vi "LiveMode.vi"() -> ()   [LabVIEW 2019]
uses:
  Data/GetPixelData16.vi
panel:
  in  "Centre AOI":bool
  in  "AOI Width":i64=2560
  in  "AOI Height":i64=2160
  out "Ready":bool
  in  "Run":bool
  in  "error":errorcluster
  out "Pixel Encoding":string
  out "Intensity Graph":u16[][](graph)
  out "AOIStride":i64
  in  "PreAmp":string(combo)="16-bit (low noise & high well capacity)"
  out "PixelData":u16[](array[numeric])
  out "ByteData":u8[](array[numeric])
  in  "ExposureTime":dbl=0.1
  out "ImageSizeBytes":i64
  out "Handle":i32
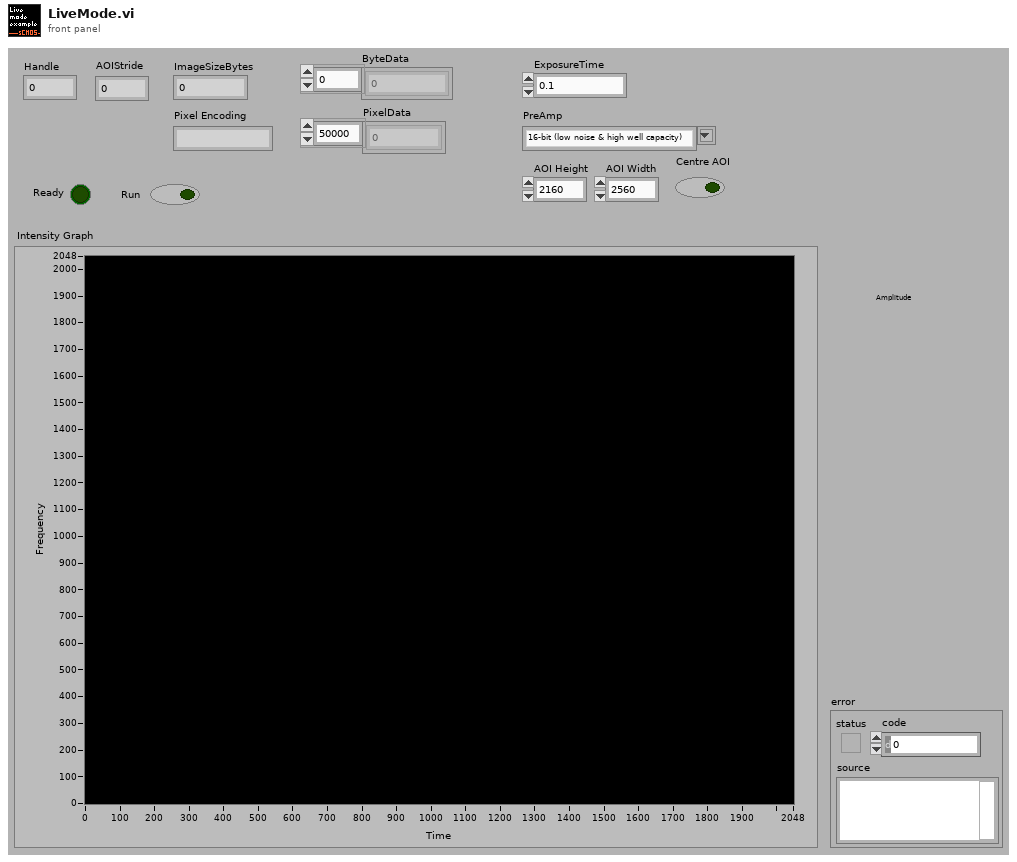
[diagram p1: front panel]
types:
  T1 = enum8{"Enabled", "Disabled", "Disabled and Grayed Out"}
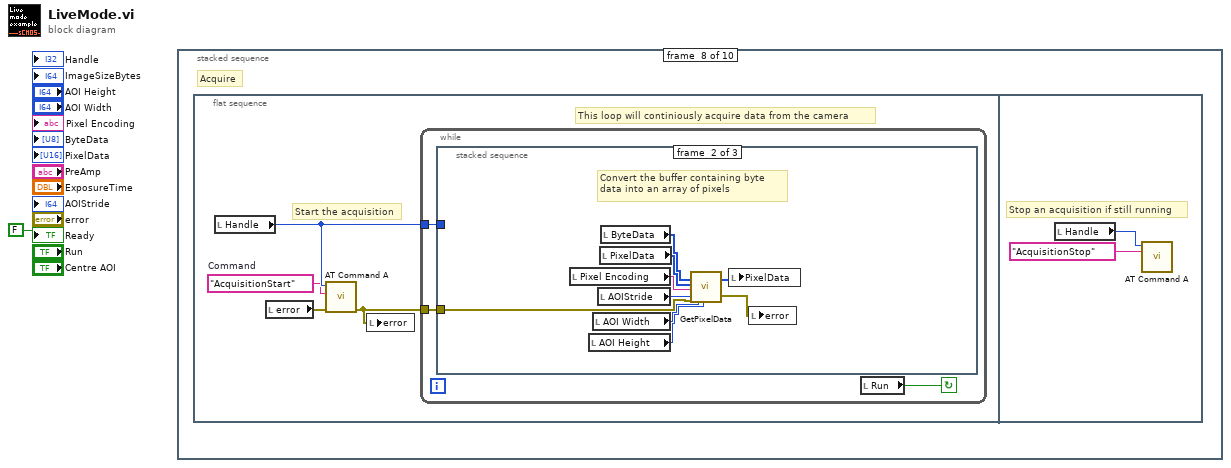
[diagram p0: block diagram]
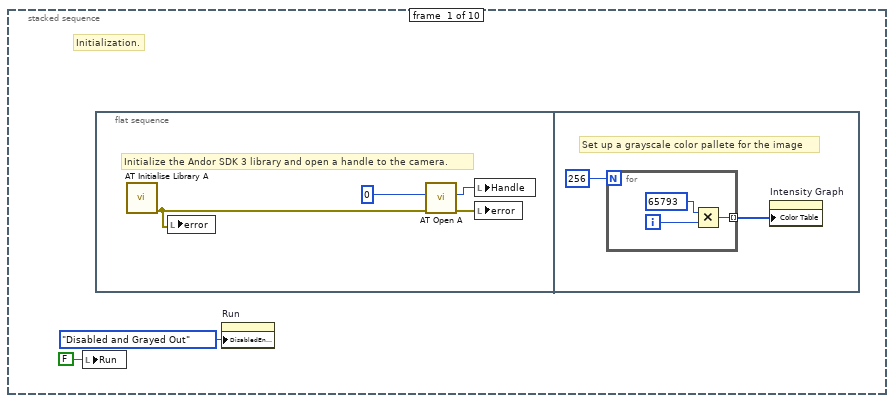
[diagram p2: hidden frame]
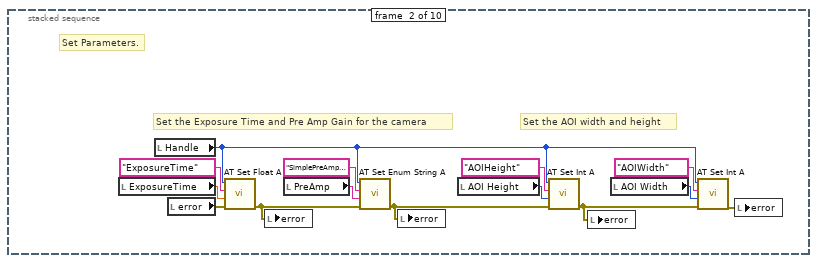
[diagram p3: hidden frame]
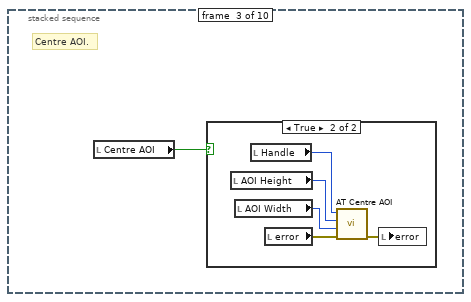
[diagram p4: hidden frame]
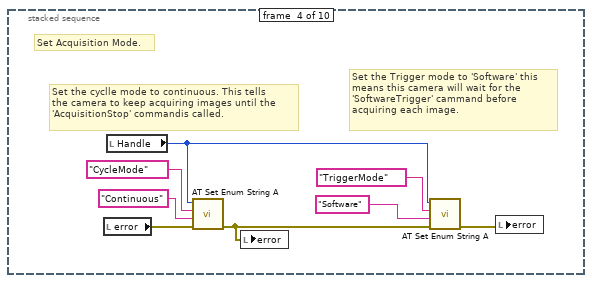
[diagram p6: hidden frame]
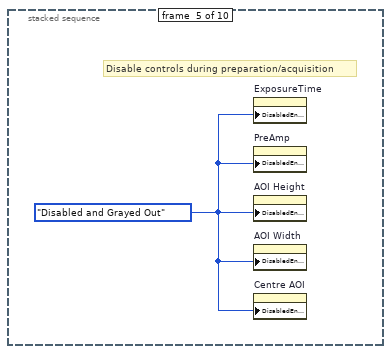
[diagram p7: hidden frame]
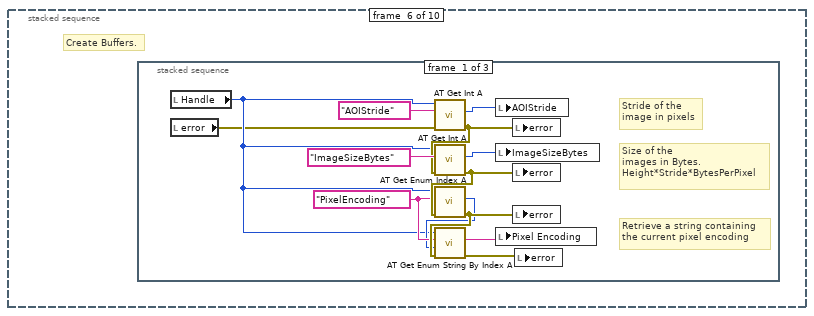
[diagram p8: hidden frame]
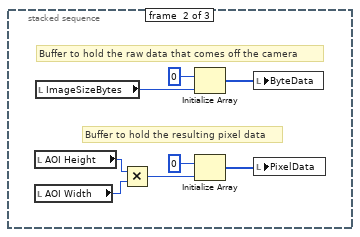
[diagram p9: hidden frame]
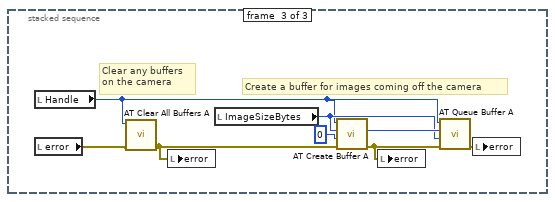
[diagram p10: hidden frame]
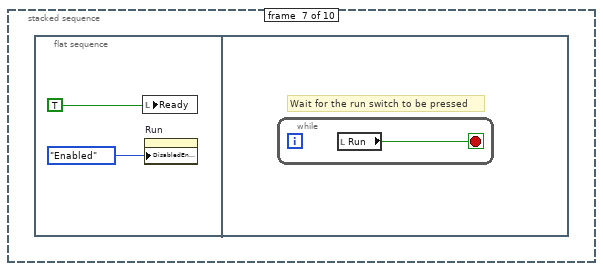
[diagram p11: hidden frame]
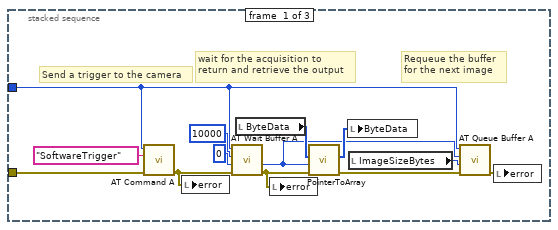
[diagram p12: hidden frame]
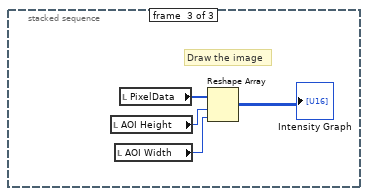
[diagram p13: hidden frame]
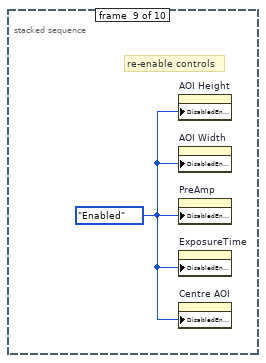
[diagram p14: hidden frame]
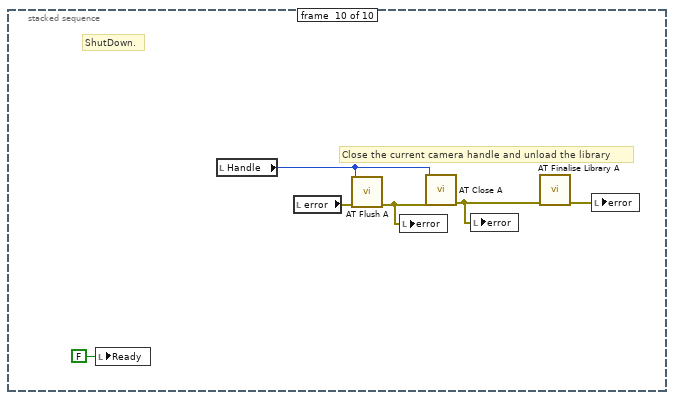
[diagram p15: hidden frame]
diagram:
  n1 = stacked-sequence {
    frame #0 {
      # "Initialization."
      n2 = local write "Run"(FALSE ("Run")) -> ()
      n3 = flat-sequence {
        frame #0 {
          # "Initialize the Andor SDK 3 library and open a handle to the camera."
          n4 = call "AT Initialise Library A.vi"() -> ("error out"=w5:errorcluster)  [unwired: 10 in, 1 out]
          n5 = local write "error"(w5) -> ()
          n6 = call "AT Open A.vi"("error in (no error)"=w5, "CameraIndex"=0) -> ("error out"=w4:errorcluster, "Handle"=w6:i32)  [unwired: 7 in, 1 out]
          n7 = local write "Handle"(w6) -> ()
          n8 = local write "error"(w4) -> ()
        }
        frame #1 {
          # "Set up a grayscale color pallete for the image"
          n9 = for {
            N: 256 -> [_]
            tunnel: [w11] -> w8 mode=indexing
            i -> [w12]
            n10 = Multiply(x=65793, y=w12) -> (x*y=w11:i32)
          }
          n11 = property on="Intensity Graph" class="IntGraph (strict)"("Color Table"=w8) -> ()  [unwired: 2 in, 2 out]
        }
      }
      n12 = property on="Run" class="Bool (strict)"("DisabledEnum"=T1."Disabled and Grayed Out" ("Disabled")) -> ()  [unwired: 2 in, 2 out]
    }
    frame #1 {
      # "Set the AOI width and height"
      # "Set the Exposure Time and Pre Amp Gain for the camera"
      # "Set Parameters."
      n13 = local read "ExposureTime"() -> (w26:dbl)
      n14 = local read "Handle"() -> (w13:i32)
      n15 = local read "error"() -> (w21:errorcluster)
      n16 = call "AT Set Float A.vi"("error in (no error)"=w21, "Value"=w26, "Feature"="ExposureTime" ("ExposureTime"), "Hndl"=w13) -> ("error out"=w24:errorcluster)  [unwired: 6 in, 1 out]
      n17 = local write "error"(w24) -> ()
      n18 = local read "PreAmp"() -> (w25:string)
      n19 = call "AT Set Enum String A.vi"("error in (no error)"=w24, "String"=w25, "Feature"="SimplePreAmpGainControl" ("SimplePreAmpGainControl"), "Handle"=w13) -> ("error out"=w20:errorcluster)  [unwired: 6 in, 1 out]
      n20 = local write "error"(w20) -> ()
      n21 = local read "AOI Height"() -> (w17:i64)
      n22 = call "AT Set Int A.vi"("error in (no error)"=w20, "Value"=w17, "Feature"="AOIHeight" ("Integer feature"), "Handle"=w13) -> ("error out"=w18:errorcluster)  [unwired: 6 in, 1 out]
      n23 = local write "error"(w18) -> ()
      n24 = local read "AOI Width"() -> (w16:i64)
      n25 = call "AT Set Int A.vi"("error in (no error)"=w18, "Value"=w16, "Feature"="AOIWidth" ("Integer feature 2"), "Handle"=w13) -> ("error out"=w19:errorcluster)  [unwired: 6 in, 1 out]
      n26 = local write "error"(w19) -> ()
    }
    frame #2 {
      # "Centre AOI."
      n27 = local read "Centre AOI"() -> (w27:bool)
      n28 = case shown="True" w27 {
        frame False {
        }
        frame True {
          n29 = local read "AOI Height"() -> (w29:i64)
          n30 = local read "AOI Width"() -> (w30:i64)
          n31 = local read "Handle"() -> (w28:i32)
          n32 = local read "error"() -> (w31:errorcluster)
          n33 = call "AT Centre AOI.vi"("error in (no error)"=w31, "AOI Width"=w30, "AOI Height"=w29, "Handle"=w28) -> ("error out"=w32:errorcluster)  [unwired: 7 in]
          n34 = local write "error"(w32) -> ()
        }
      }
    }
    frame #3 {
      # "Set the Trigger mode to 'Software' this \nmeans this camera will wait for the \n'SoftwareTrigger' cammand before \nacquiring each image."
      # "Set the cyclle mode to continuous. This tells \nthe camera to keep acquiring images until the \n'AcquisitionStop' commandis called."
      # "Set Acquisition Mode."
      n35 = local read "error"() -> (w38:errorcluster)
      n36 = local read "Handle"() -> (w35:i32)
      n37 = call "AT Set Enum String A.vi"("error in (no error)"=w38, "String"="Continuous", "Feature"="CycleMode" ("Enum feature"), "Handle"=w35) -> ("error out"=w37:errorcluster)  [unwired: 6 in, 1 out]
      n38 = local write "error"(w37) -> ()
      n39 = call "AT Set Enum String A.vi"("error in (no error)"=w37, "String"="Software", "Feature"="TriggerMode" ("Enum feature"), "Handle"=w35) -> ("error out"=w33:errorcluster)  [unwired: 6 in, 1 out]
      n40 = local write "error"(w33) -> ()
    }
    frame #4 {
      w41 = T1."Disabled and Grayed Out" ("Disabled")
      # "Disable controls during preparation/acquisition"
      n41 = property on="ExposureTime" class="DigNum (strict)"("DisabledEnum"=w41) -> ()  [unwired: 2 in, 2 out]
      n42 = property on="PreAmp" class="CmbBox"("DisabledEnum"=w41) -> ()  [unwired: 2 in, 2 out]
      n43 = property on="AOI Height" class="DigNum (strict)"("DisabledEnum"=w41) -> ()  [unwired: 2 in, 2 out]
      n44 = property on="AOI Width" class="DigNum (strict)"("DisabledEnum"=w41) -> ()  [unwired: 2 in, 2 out]
      n45 = property on="Centre AOI" class="Bool (strict)"("DisabledEnum"=w41) -> ()  [unwired: 2 in, 2 out]
    }
    frame #5 {
      # "Create Buffers."
      n46 = stacked-sequence {
        frame #0 {
          w47 = "PixelEncoding" ("Enum feature")
          # "Retrieve a string containing \nthe current pixel encoding"
          # "Stride of the\nimage in pixels"
          # "Size of the\nimages in Bytes.\nHeight*Stride*BytesPerPixel"
          n47 = local read "Handle"() -> (w43:i32)
          n48 = local read "error"() -> (w42:errorcluster)
          n49 = call "AT Get Int A.vi"("error in (no error)"=w42, "Feature"="AOIStride" ("Integer feature"), "Handle"=w43) -> ("error out"=w50:errorcluster, "Value"=w54:i64)  [unwired: 6 in, 1 out]
          n50 = call "AT Get Int A.vi"("error in (no error)"=w50, "Feature"="ImageSizeBytes" ("Integer feature"), "Handle"=w43) -> ("error out"=w49:errorcluster, "Value"=w53:i64)  [unwired: 6 in, 1 out]
          n51 = call "AT Get Enum Index A.vi"("error in (no error)"=w49, "Feature"=w47, "Handle"=w43) -> ("error out"=w48:errorcluster, "Value"=w46:i32)  [unwired: 6 in, 1 out]
          n52 = call "AT Get Enum String By Index A.vi"("error in (no error)"=w48, "Index"=w46, "Feature"=w47, "Handle"=w43) -> ("error out"=w44:errorcluster, "String"=w45:string)  [unwired: 5 in, 1 out]
          n53 = local write "AOIStride"(w54) -> ()
          n54 = local write "ImageSizeBytes"(w53) -> ()
          n55 = local write "Pixel Encoding"(w45) -> ()
          n56 = local write "error"(w50) -> ()
          n57 = local write "error"(w49) -> ()
          n58 = local write "error"(w48) -> ()
          n59 = local write "error"(w44) -> ()
        }
        frame #1 {
          # "Buffer to hold the resulting pixel data"
          # "Buffer to hold the raw data that comes off the camera"
          n60 = local read "AOI Height"() -> (w60:i64)
          n61 = local read "AOI Width"() -> (w61:i64)
          n62 = local read "ImageSizeBytes"() -> (w56:i64)
          n63 = Multiply(x=w60, y=w61) -> (x*y=w55:i64)
          n64 = Initialize Array(u8 0, w56) -> (w58:u8[])
          n65 = Initialize Array(i64 0, w55) -> (w59:i64[])
          n66 = local write "ByteData"(w58) -> ()
          n67 = local write "PixelData"(w59) -> ()
        }
        frame #2 {
          # "Clear any buffers \non the camera"
          # "Create a buffer for images coming off the camera"
          n68 = local read "Handle"() -> (w63:i32)
          n69 = local read "error"() -> (w65:errorcluster)
          n70 = call "AT Clear All Buffers A.vi"("error in (no error)"=w65, "Handle"=w63) -> ("error out"=w64:errorcluster)  [unwired: 8 in, 1 out]
          n71 = local write "error"(w64) -> ()
          n72 = local read "ImageSizeBytes"() -> (w67:i64)
          n73 = call "AT Create Buffer A.vi"("error in (no error)"=w64, "Buffer"=0 ("Size"), "Size"=w67, "Handle"=w63) -> ("error out"=w69:errorcluster, "Buffer out"=w70:u64)  [unwired: 5 in, 1 out]
          n74 = local write "error"(w69) -> ()
          n75 = call "AT Queue Buffer A.vi"("error in (no error)"=w69, "PtrSize"=w67, "Ptr"=w70, "Handle"=w63) -> ("error out"=w66:errorcluster)  [unwired: 6 in, 1 out]
          n76 = local write "error"(w66) -> ()
        }
      }
    }
    frame #6 {
      n77 = flat-sequence {
        frame #0 {
          n78 = local write "Ready"(TRUE ("Ready")) -> ()
          n79 = property on="Run" class="Bool (strict)"("DisabledEnum"=T1."Enabled" ("Disabled")) -> ()  [unwired: 2 in, 2 out]
        }
        frame #1 {
          # "Wait for the run switch to be pressed"
          n80 = while {
            stop <- w73 stop-if-true
            n81 = local read "Run"() -> (w73:bool)
          }
        }
      }
    }
    frame #7 {
      # "Acquire"
      n82 = flat-sequence {
        frame #0 {
          w75 = "AcquisitionStart"  # Command
          # "This loop will continiously acquire data from the camera"
          # "Start the acquisition"
          n83 = local read "Handle"() -> (w77:i32)
          n84 = local read "error"() -> (w76:errorcluster)
          n85 = call "AT Command A.vi"("error in (no error)"=w76, "Feature"=w75, "Handle"=w77) -> ("error out"=w74:errorcluster)  [unwired: 7 in, 1 out]
          n86 = local write "error"(w74) -> ()
          n87 = while {
            tunnel: w77 -> [w79]
            tunnel: w74 -> [w80]
            stop <- w78 continue-if-true
            n88 = stacked-sequence {
              tunnel: w80 -> [w87 w94 _]
              tunnel: w79 -> [w88 _ _]
              frame #0 {
                # "Requeue the buffer\nfor the next image"
                # "Send a trigger to the camera"
                # "wait for the acquisition to \nreturn and retrieve the output"
                n89 = call "AT Command A.vi"("error in (no error)"=w87, "Feature"="SoftwareTrigger" ("Command"), "Handle"=w88) -> ("error out"=w86:errorcluster)  [unwired: 7 in, 1 out]
                n90 = local write "error"(w86) -> ()
                n91 = call "AT Wait Buffer A.vi"("error in (no error)"=w86, "Input buffer"=u32 0, "Timeout"=u32 10000, "Handle"=w88) -> ("error out"=w85:errorcluster, "Output buffer"=w81:u64)  [unwired: 4 in, 2 out]
                n92 = local read "ByteData"() -> (w83:u8[])
                n93 = local write "error"(w85) -> ()
                n94 = call "PointerToArray.vi"("error in (no error)"=w85, "Pointer In"=w81, "Array in"=w83) -> ("error out"=w84:errorcluster, "Array out"=w82:u8[])  [unwired: 7 in]
                n95 = local write "ByteData"(w82) -> ()
                n96 = local read "ImageSizeBytes"() -> (w93:i64)
                n97 = call "AT Queue Buffer A.vi"("error in (no error)"=w84, "PtrSize"=w93, "Ptr"=w81, "Handle"=w88) -> ("error out"=w90:errorcluster)  [unwired: 6 in, 1 out]
                n98 = local write "error"(w90) -> ()
              }
              frame #1 {
                # "Convert the buffer containing byte \ndata into an array of pixels"
                n99 = local read "Pixel Encoding"() -> (w100:string)
                n100 = local read "AOI Height"() -> (w97:i64)
                n101 = local read "AOI Width"() -> (w98:i64)
                n102 = local read "AOIStride"() -> (w101:i64)
                n103 = local read "PixelData"() -> (w99:u16[])
                n104 = local read "ByteData"() -> (w95:u8[])
                n105 = call-poly "GetPixelData.vi"("Input buffer"=w95, "Output buffer in"=w99, "Pixel Encoding"=w100, "Stride"=w101, "error in (no error)"=w94, "Width"=w98, "Height"=w97) -> ("Output buffer out"=w102:u16[], "error out"=w96:errorcluster)  [unwired: 10 in, 1 out]
                n106 = local write "PixelData"(w102) -> ()
                n107 = local write "error"(w96) -> ()
              }
              frame #2 {
                # "Draw the image"
                n108 = local read "AOI Height"() -> (w105:i64)
                n109 = local read "AOI Width"() -> (w104:i64)
                n110 = local read "PixelData"() -> (w106:u16[])
                n111 = Reshape Array(w106, w105, w104) -> (→"Intensity Graph":u16[][])
              }
            }
            n112 = local read "Run"() -> (w78:bool)
          }
        }
        frame #1 {
          # "Stop an acquisition if still running"
          n113 = local read "Handle"() -> (w108:i32)
          n114 = call "AT Command A.vi"("Feature"="AcquisitionStop" ("Command"), "Handle"=w108) -> ()  [unwired: 8 in, 2 out]
        }
      }
    }
    frame #8 {
      w109 = T1."Enabled" ("Disabled")
      # "re-enable controls"
      n115 = property on="AOI Height" class="DigNum (strict)"("DisabledEnum"=w109) -> ()  [unwired: 2 in, 2 out]
      n116 = property on="AOI Width" class="DigNum (strict)"("DisabledEnum"=w109) -> ()  [unwired: 2 in, 2 out]
      n117 = property on="PreAmp" class="CmbBox"("DisabledEnum"=w109) -> ()  [unwired: 2 in, 2 out]
      n118 = property on="ExposureTime" class="DigNum (strict)"("DisabledEnum"=w109) -> ()  [unwired: 2 in, 2 out]
      n119 = property on="Centre AOI" class="Bool (strict)"("DisabledEnum"=w109) -> ()  [unwired: 2 in, 2 out]
    }
    frame #9 {
      # "Close the current camera handle and unload the library"
      # "ShutDown."
      n120 = local write "Ready"(FALSE ("Ready")) -> ()
      n121 = local read "Handle"() -> (w110:i32)
      n122 = local read "error"() -> (w113:errorcluster)
      n123 = call "AT Flush A.vi"("error in (no error)"=w113, "Handle"=w110) -> ("error out"=w114:errorcluster)  [unwired: 8 in, 1 out]
      n124 = local write "error"(w114) -> ()
      n125 = call "AT Close A.vi"("error in (no error)"=w114, "Handle"=w110) -> ("error out"=w115:errorcluster)  [unwired: 8 in, 1 out]
      n126 = local write "error"(w115) -> ()
      n127 = call "AT Finalise Library A.vi"("error in (no error)"=w115) -> ("error out"=w111:errorcluster)  [unwired: 9 in, 1 out]
      n128 = local write "error"(w111) -> ()
    }
  }
  "Ready" <- FALSE ("Ready")
